vi "FP_Get Monitor WorkSpace.vi"(3 "Monitor #":u16) -> (1 "Disp.WkSpace Out":T1)   [LabVIEW 2016]
uses:
  <vilib>/Utility/miscctls.llb/LVRectTypeDef.ctl
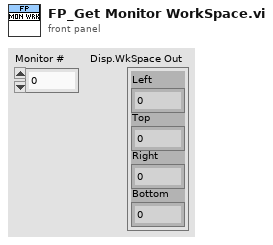
[diagram p1: front panel]
types:
  T1 = typedef "LVRectTypeDef.ctl" = cluster{"Left":i16, "Top":i16, "Right":i16, "Bottom":i16}
  T2 = typedef "LVAllMonitorsDisplayTypeDef.ctl" = cluster{"Bounds":cluster{"Left":i16, "Top":i16, "Right":i16, "Bottom":i16}, "Depth":i16}[]
  T3 = cluster{"Bounds":cluster{"Left":i16, "Top":i16, "Right":i16, "Bottom":i16}, "Depth":i16}
  T4 = cluster{"Left":i16, "Top":i16, "Right":i16, "Bottom":i16}
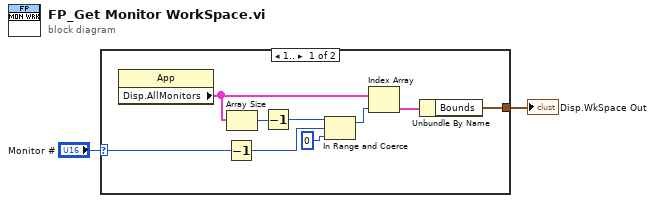
[diagram p0: block diagram]
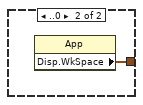
[diagram p2: hidden frame]
diagram:
  n1 = case shown="1.." "Monitor #" {
    selector: "Monitor #" -> [w8 _]
    tunnel: [w3 w12] -> w2
    frame 1.. {
      n2 = property class="App"() -> ("Disp.AllMonitors"=w6:T2)  [unwired: 2 in, 2 out]
      n3 = Decrement(x=w8) -> (x-1=w7:u16)
      n4 = Array Size(array=w6) -> (size(s)=w11:i32)
      n5 = Decrement(x=w11) -> (x-1=w10:i32)
      n6 = In Range and Coerce(upper limit=w10, x=w7, lower limit=0) -> (coerced(x)=w5:i32)  [unwired: 1 out]
      n7 = Index Array(array=w6, index=w5) -> (element=w4:T3)
      n8 = Unbundle By Name(w4) -> ("Bounds"=w3:T4)
    }
    frame ..0 {
      n9 = property class="App"() -> ("Disp.WkSpace"=w12:T1)  [unwired: 2 in, 2 out]
    }
  }
  "Disp.WkSpace Out" <- w2
